vi "MPM_Get_Logging_Data_Point.vi"(8 "error in (no error)":errorcluster, 11 ".NET Reference in":refnum<k24>) -> (0 "error out":errorcluster, 2 "count out":i32, 3 "Reference out":refnum<k24>)   [LabVIEW 2017]
uses:
  C:/Users/Ssantec_Test/Documents/Instrument_DLL_Sample_Labview_20220902_Ver1.2.2/DLL/x86/InstrumentDLL.dll
  DLL/x86/InstrumentDLL.dll
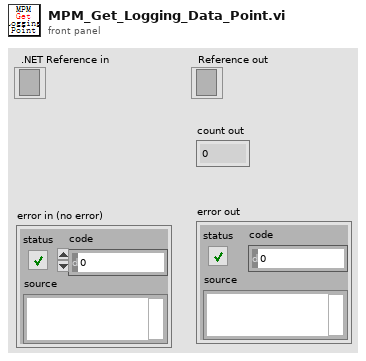
[diagram p1: front panel]
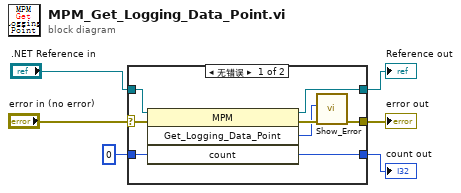
[diagram p0: block diagram]
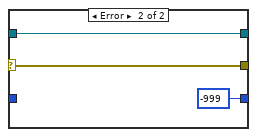
[diagram p2: hidden frame]
diagram:
  n1 = case shown="无错误" "error in (no error)" {
    selector: "error in (no error)" -> [w7 w16]
    tunnel: [w14 -999 ("count")] -> w6
    tunnel: ".NET Reference in" -> [w13 w17]
    tunnel: [w12 w17] -> w4
    tunnel: 0 ("count") -> [w11 _]
    tunnel: [w8 w16] -> w2
    frame No Error {
      n2 = invoke class="MPM" method="Get_Logging_Data_Point"(reference=w13, error in=w7, "count"=w11) -> (reference out=w12:refnum<k24>, error out=w10:errorcluster, "Get_Logging_Data_Point"=w9:i32, "count"=w14:i32)  [unwired: 1 in]
      n3 = call "Show_Error.vi"("error in (no error)"=w10, "Error"=w9) -> ("error out"=w8:errorcluster)  [unwired: 9 in]
    }
    frame Error {
    }
  }
  "count out" <- w6
  "Reference out" <- w4
  "error out" <- w2
